vi "Renew Controls Attribute.vi"(8 "error in (no error)":errorcluster, 10 "Control Refs":refnum<vi>[](array[refnum]), 11 "ScriptsDialogConfiguration in":refnum<class "ScriptsDialogConfiguration.lvclass">) -> (0 "error out":errorcluster, 3 "ScriptsDialogConfiguration out":refnum<class "ScriptsDialogConfiguration.lvclass">)   [LabVIEW 2015, in "ScriptsDialogConfiguration.lvclass"]
uses:
  ScriptsDialogConfiguration.lvclass
  UIConfiguration/UIConfiguration.lvclass/UIConfiguration.ctl
  UIConfiguration/UIConfiguration.lvclass
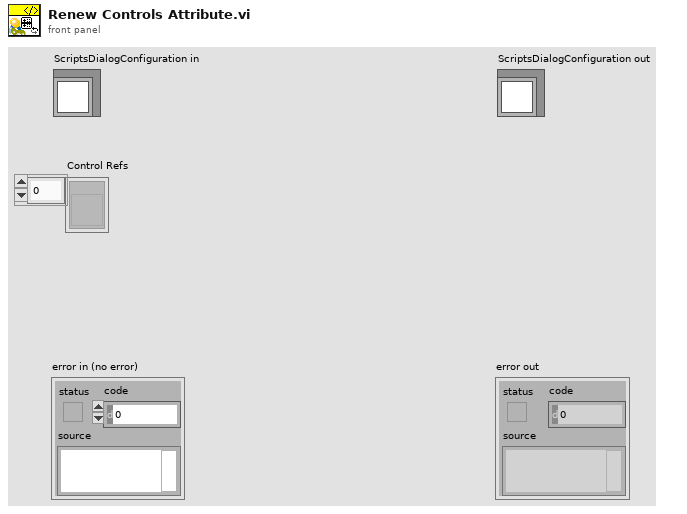
[diagram p1: front panel]
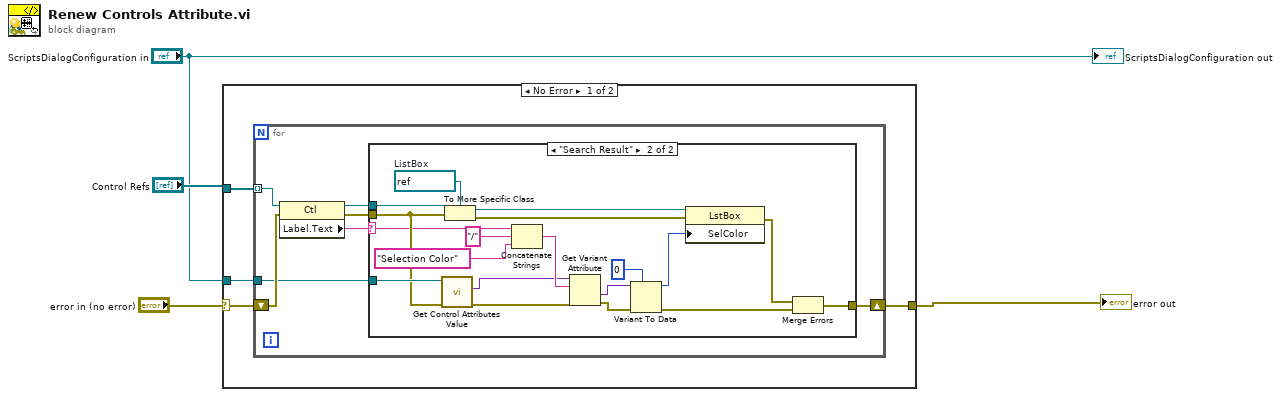
[diagram p0: block diagram]
diagram:
  n1 = case shown="No Error" "error in (no error)" {
    selector: "error in (no error)" -> [w7 w36]
    tunnel: "Control Refs" -> [w8 _]
    tunnel: [w6 w36] -> w2
    tunnel: "ScriptsDialogConfiguration in" -> [w5 _]
    frame No Error {
      n2 = for {
        tunnel: w8 -> [w15] mode=indexing
        tunnel: w5 -> [w10]
        shift-right: [w9] -> w6
        shift-left: w7 -> [w14]
        n3 = property class="Ctl"(reference=w15, error in=w14) -> (reference out=w11:refnum<vi>, error out=w12:errorcluster, "Label.Text"=w13:string)
        n4 = case shown="\"Search Result\"" w13 {
          selector: w13 -> [_ w29]
          tunnel: w12 -> [w16 w30]
          tunnel: w11 -> [_ w35]
          tunnel: w10 -> [_ w31]
          tunnel: [w16 w17] -> w9
          frame Default {
          }
          frame "Search Result" {
            w34 = refnum<vi> refnum  # ListBox
            n5 = call "Get Control Attributes Value.vi"("error in (no error)"=w30, "UIConfiguration in"=w31) -> ("error out"=w24:errorcluster, "AttributesValue"=w25:variant)  [unwired: 7 in, 1 out]
            n6 = To More Specific Class(target class=w34, reference=w35, error in=w30) -> (specific class reference=w33:refnum<vi>, error out=w32:errorcluster)
            n7 = Concatenate Strings(w29, "/" ("string"), "Selection Color" ("string")) -> (w26:string)
            n8 = Get Variant Attribute(Variant=w25, name=w26, error in=w24) -> (value=w23:variant, error out=w22:errorcluster)  [unwired: 1 in, 2 out]
            n9 = Variant To Data(error in=w22, type=u32 0 ("Selection Color"), Variant=w23) -> (data=w20:u32, error out=w18:errorcluster)
            n10 = property class="LstBox"(reference=w33, error in=w32, "SelColor"=w20) -> (error out=w19:errorcluster)  [unwired: 1 out]
            n11 = Merge Errors(w19, w18) -> (w17:errorcluster)
          }
        }
      }
    }
    frame Error {
    }
  }
  "error out" <- w2
  "ScriptsDialogConfiguration out" <- "ScriptsDialogConfiguration in"
